vi "runSalMonitor.vi"(8 "error in (no error)":errorcluster, 9 "pathOfOutput":path, 10 "pathOfSalMonitor":path, 11 "SalProcess in":refnum<class "SalProcess.lvclass">) -> (0 "error out":errorcluster, 3 "SalProcess out":refnum<class "SalProcess.lvclass">)   [LabVIEW 2018, in "SalProcess.lvclass"]
doc: "Run the SAL monitor in the background."
uses:
  SalProcess.lvclass
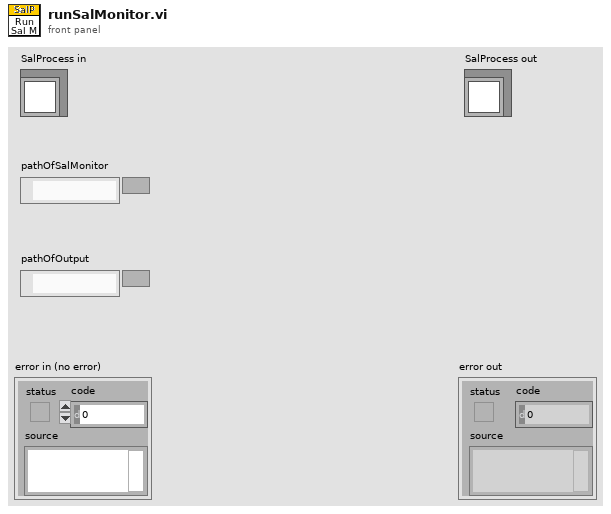
[diagram p1: front panel]
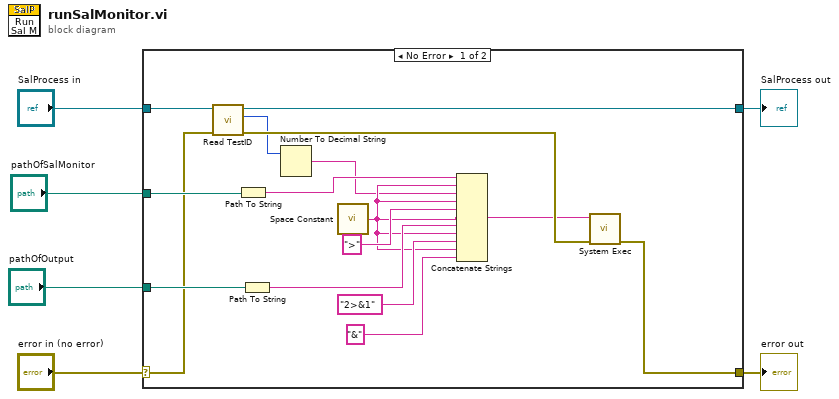
[diagram p0: block diagram]
diagram:
  n1 = case shown="No Error" "error in (no error)" {
    selector: "error in (no error)" -> [w13 w24]
    tunnel: [w21 w24] -> w5
    tunnel: [w14 w23] -> w3
    tunnel: "SalProcess in" -> [w15 w23]
    tunnel: "pathOfSalMonitor" -> [w22 _]
    tunnel: "pathOfOutput" -> [w20 _]
    frame No Error {
      n2 = call "Read TestID.vi"("error in (no error)"=w13, "SalProcess in"=w15) -> ("error out"=w12:errorcluster, "TestID"=w10:i32, "SalProcess out"=w14:refnum<class "SalProcess.lvclass">)  [unwired: 7 in]
      n3 = Path To String(path=w22) -> (string=w9:string)
      n4 = Path To String(path=w20) -> (string=w18:string)
      n5 = Number To Decimal String(number=w10) -> (decimal integer string=w7:string)  [unwired: 1 in]
      n6 = call <vilib>:"Space Constant.vi"() -> ("String"=w8:string)
      n7 = Concatenate Strings(w9, w8, w7, w8, ">", w8, w18, w8, "2>&1", w8, "&") -> (w11:string)
      n8 = call <vilib>:"System Exec.vi"("error in (no error)"=w12, "command line"=w11) -> ("error out"=w21:errorcluster)  [unwired: 6 in, 3 out]
    }
    frame Error {
    }
  }
  "error out" <- w5
  "SalProcess out" <- w3
